vi "Grab.vi"(8 "error in (no error)":errorcluster, 10 "Grab Toggle?":bool, 11 "Hatch in":refnum<class "Hatch.lvclass">) -> (0 "error out":errorcluster, 2 "Solenoid On?":bool, 3 "Hatch out":refnum<class "Hatch.lvclass">)   [LabVIEW 2018, in "Hatch.lvlib" / "Hatch.lvclass"]
doc: "Use this VI to grab or releas a hatch"
uses:
  Hatch.lvclass
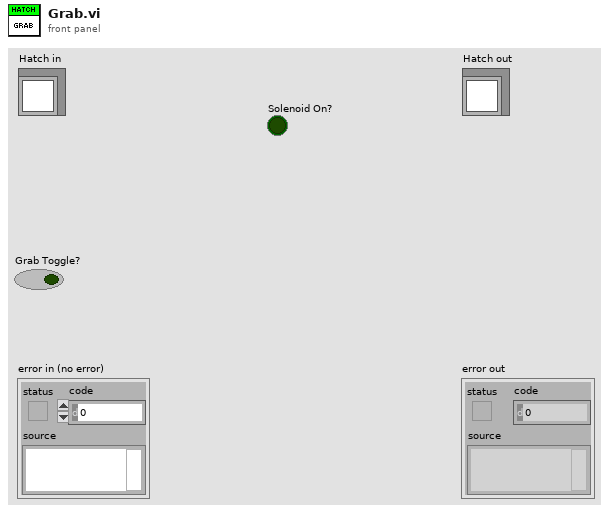
[diagram p1: front panel]
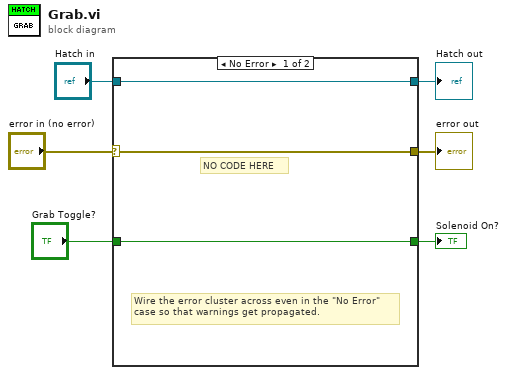
[diagram p0: block diagram]
diagram:
  n1 = case shown="No Error" "error in (no error)" {
    selector: "error in (no error)" -> [w8 w11]
    tunnel: [w8 w11] -> w5
    tunnel: [w9 w10] -> w3
    tunnel: "Hatch in" -> [w9 w10]
    tunnel: [w7 _] -> w2
    tunnel: "Grab Toggle?" -> [w7 _]
    frame No Error {
      # "NO CODE HERE"
      # "Wire the error cluster across even in the \"No Error\"\ncase so that warnings get propagated."
    }
    frame Error {
    }
  }
  "error out" <- w5
  "Hatch out" <- w3
  "Solenoid On?" <- w2
